vi "setTransmission.vi"(1 "SetTransmission":i16=1 min=0 max=100, 2 "VISA resource name":refnum<visa-resource-name>) -> ()   [LabVIEW 2013]
panel:
  out "hex integer string 2":string
  out "EnergyCommand 2":string
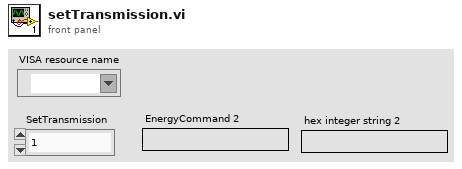
[diagram p1: front panel]
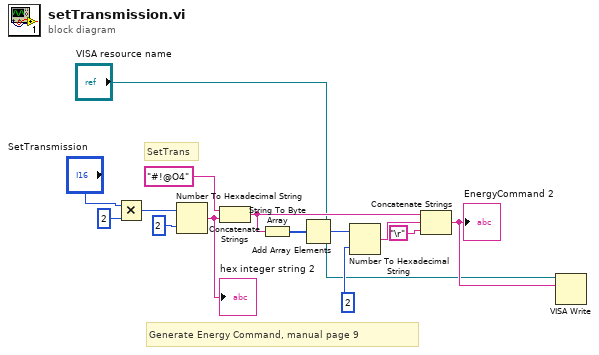
[diagram p0: block diagram]
diagram:
  # "Generate Energy Command, manual page 9"
  # "SetTrans"
  n1 = Multiply(x="SetTransmission", y=2) -> (x*y=w14:i32)
  n2 = Number To Hexadecimal String(1:i16 2 ("width (-)"), 2:w14) -> (0:w6:string)
  "hex integer string 2" <- w6
  n3 = Concatenate Strings("#!@O4" ("string"), w6) -> (w10:string)
  n4 = String To Byte Array(string=w10) -> (unsigned byte array=w7:u8[])
  n5 = Add Array Elements(numeric array=w7) -> (sum=w8:u8)
  n6 = Number To Hexadecimal String(1:i16 2 ("width (-)"), 2:w8) -> (0:w11:string)
  n7 = Concatenate Strings(w10, w11, "\r") -> (w2:string)
  "EnergyCommand 2" <- w2
  n8 = VISA Write(VISA resource name="VISA resource name", write buffer=w2) -> ()  [unwired: 1 in, 3 out]
